vi "ApertureTime_StdDev.vi"() -> ()   [LabVIEW 2019]
panel:
  out "Standard Deviation vs Aperture Time":T1(graph)={"Standard Deviation (Ohm)"=[0.0166666, 0.033333, 0.05, 0.0666666, 0.0833333, 0.1, 0.2], "Aperture Time (s)"=[1.75576e-07, 1.57484e-07, 1.19793e-07, 1.12763e-07, 1.07534e-07, 1.00072e-07, 9.4697e-08]}
  in  "Test Time (s)":dbl[](array[numeric])=[31.757, 61.714, 91.658, 121.614, 151.558, 181.508, 361.218] format="%#_6p"
  in  "Standard Deviation (Ohm)":dbl[](array[numeric])=[2.2855e-07, 1.30614e-07, 1.1847e-07, 1.08107e-07, 1.00751e-07, 98.626, 88.859] format="%#_6p"
  in  "DMM and SMU Aperture Time (s)":dbl[](array[numeric])=[0.0166666, 0.033333, 0.05, 0.0666666, 0.0833333, 0.1, 0.2] format="%#_6p"
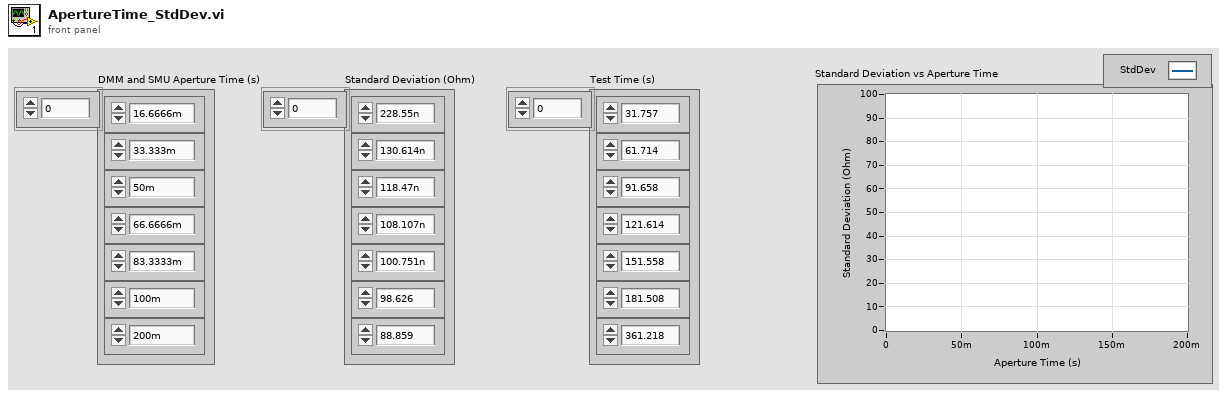
[diagram p1: front panel]
types:
  T1 = cluster{"Standard Deviation (Ohm)":dbl[], "Aperture Time (s)":dbl[]}
  T2 = cluster{"DMM and SMU Aperture Time (s)":dbl[], "Standard Deviation (Ohm)":dbl[]}
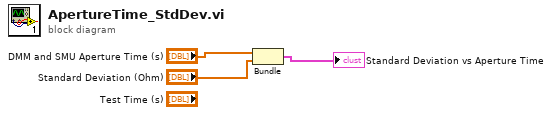
[diagram p0: block diagram]
diagram:
  n1 = Bundle("DMM and SMU Aperture Time (s)"="DMM and SMU Aperture Time (s)", "Standard Deviation (Ohm)"="Standard Deviation (Ohm)") -> (→"Standard Deviation vs Aperture Time":T2)  [unwired: 1 in]
